vi "Index Array__ogtk.vi"(8 "error in (no error)":errorcluster, 9 "Indices (>=1D)":u32[](array[numeric]), 10 "Index (1D)":u32, 11 "MultiD Array":variant) -> (0 "error out":errorcluster, 2 "Array Element":variant)   [LabVIEW 2016]
doc: "Returns the element of a MultiD array at given indices. Inefficient for large arrays."
panel:
  # "[OpenG VI Tags] ***Do Not Remove***"
  # "Index Array.vi\n\nReturns the element of a MultiD array at given indices. Inefficient for large ar\n\nPlease visit http://www.OpenG.org to learn about the\nOpen Source LabVIEW software movement.\n\nNOTICE -- YOU MUST LEAVE THIS NOTICE IN PLACE.  PER THE TERMS OF THE LICENSE BELOW, YOU MAY SUBLICENSE THIS SOFTWARE \nIN ANY WAY THAT DOES NOT CONFLICT WITH THIS LICENSE.\n\n### BSD License (http://www.opensource.org/licenses/bsd-license.php) Begin ###\n \nCopyright (c) 2002, Jean-Pierre Drolet <drolet_jp@hotmail.com>\nCopyright (c) 2002-2006, Jim Kring <jim@jimkring.com>\n\nAll rights reserved.\n\nRedistribution and use in source and binary forms, with or without modification, are permitted provided that the following conditions are met:\n\n    * Redistributions of source code must retain the above copyright notice, this list of conditions and the following disclaimer.\n    * Redistributions in binary form must reproduce the above copyright notice, this list of conditions and the following disclaimer in the \n       documentation and/or other materials provided with the distribution.\n    * Neither the name of SciWare, James Kring, Inc., nor the names of its contributors may be used to endorse or promote products derived \n       from this software without specific prior written permission.\n\nTHIS SOFTWARE IS PROVIDED BY THE COPYRIGHT HOLDERS AND CONTRIBUTORS \"AS IS\" AND ANY EXPRESS OR IMPLIED WARRANTIES, \nINCLUDING, BUT NOT LIMITED TO, THE IMPLIED WARRANTIES OF MERCHANTABILITY AND FITNESS FOR A PARTICULAR PURPOSE ARE \nDISCLAIMED. IN NO EVENT SHALL THE COPYRIGHT OWNER OR CONTRIBUTORS BE LIABLE FOR ANY DIRECT, INDIRECT, INCIDENTAL,\n SPECIAL, EXEMPLARY, OR CONSEQUENTIAL DAMAGES (INCLUDING, BUT NOT LIMITED TO, PROCUREMENT OF SUBSTITUTE GOODS OR \nSERVICES; LOSS OF USE, DATA, OR PROFITS; OR BUSINESS INTERRUPTION) HOWEVER CAUSED AND ON ANY THEORY OF LIABILITY, \nWHETHER IN CONTRACT, STRICT LIABILITY, OR TORT (INCLUDING NEGLIGENCE OR OTHERWISE) ARISING IN ANY WAY OUT OF THE USE \nOF THIS SOFTWARE, EVEN IF ADVISED OF THE POSSIBILITY OF SUCH DAMAGE.\n\n### BSD License End ###"
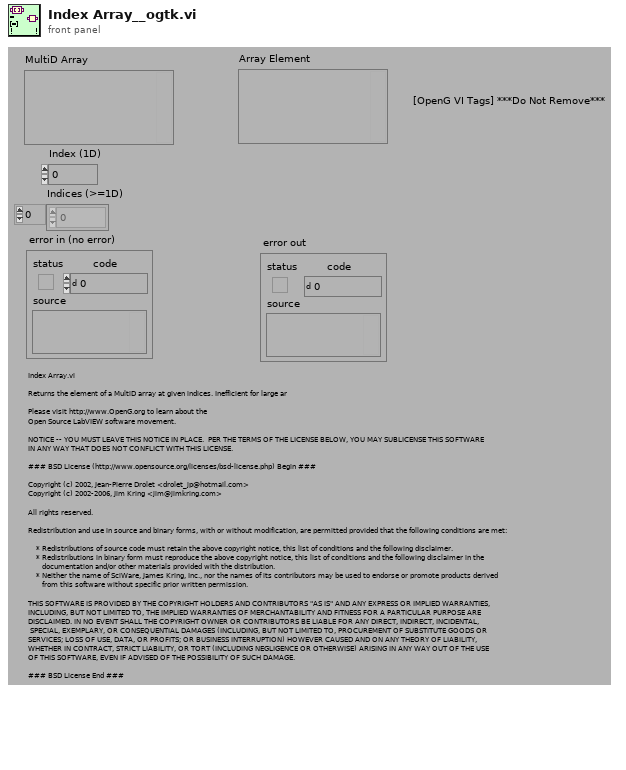
[diagram p1: front panel]
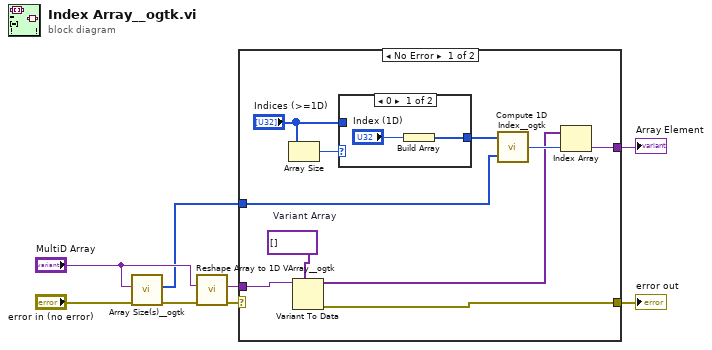
[diagram p0: block diagram]
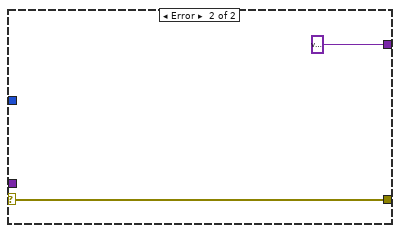
[diagram p3: hidden frame]
diagram:
  n1 = call <userlib>:"Array Size(s)__ogtk.vi"("error in (no error)"="error in (no error)", "Array"="MultiD Array") -> ("error out"=w5:errorcluster, "Size(s)"=w2:u32[])  [unwired: 7 in, 1 out]
  n2 = call <userlib>:"Reshape Array to 1D VArray__ogtk.vi"("error in (no error)"=w5, "MultiD Array"="MultiD Array") -> ("error out"=w7:errorcluster, "1D VArray"=w6:variant)  [unwired: 7 in, 1 out]
  n3 = case shown="No Error" w7 {
    selector: w7 -> [_ w23]
    tunnel: [w9 w23] -> w8
    tunnel: w6 -> [w18 _]
    tunnel: w2 -> [w14 _]
    tunnel: [w10 variant ("MultiD Array")] -> w1
    frame No Error {
      w17 = variant[] []  # Variant Array
      n4 = Array Size(array="Indices (>=1D)") -> (size(s)=w16:i32)
      n5 = Variant To Data(type=w17, Variant=w18) -> (data=w11:variant[], error out=w9:errorcluster)  [unwired: 1 in]
      n6 = case shown="0" w16 {
        tunnel: [w19 w21] -> w13
        tunnel: "Indices (>=1D)" -> [_ w21]
        frame 0 {
          n7 = Build Array("Index (1D)") -> (w19:u32[])
        }
        frame Default {
        }
      }
      n8 = call <userlib>:"Compute 1D Index__ogtk.vi"("Size(s)"=w14, "Indices"=w13) -> ("1D Index"=w12:i32)
      n9 = Index Array(array=w11, index=w12) -> (element=w10:variant)
    }
    frame Error {
    }
  }
  "error out" <- w8
  "Array Element" <- w1
